vi "isr_ESP32.vi"() -> (7 "SenalFuga":bool)   [LabVIEW 2019]
uses:
  <vilib>/myRIO/Instrument Drivers/Onboard IO/DIO/typedefs/DIO Reference.ctl
  <vilib>/myRIO/Common/Instrument Driver Framework/Utilities/typedefs/myRIO Generic Hardware Reference.ctl
  <vilib>/myRIO/Common/Instrument Driver Framework/Utilities/typedefs/Hardware Version Enum.ctl
  <vilib>/myRIO/Common/Instrument Driver Framework/Utilities/typedefs/myRIO v1.0 Reference.ctl
  <vilib>/myRIO/Common/Instrument Driver Framework/Utilities/typedefs/Generic FPGA Reference.ctl
  <vilib>/myRIO/Common/Instrument Driver Framework/myRIO v1.0/DIO/typedefs/DIO Channels List.ctl
  <vilib>/myRIO/Common/Instrument Driver Framework/myRIO v1.0/DIO/typedefs/DIO Channels Enum.ctl
  <vilib>/userDefined/High Color/nirio_resource_hc.ctl
  <vilib>/myRIO/Common/Instrument Driver Framework/Utilities/vis/Is FPGA Ref Available.vi
  <vilib>/myRIO/Common/Instrument Driver Framework/myRIO v1.0/DIO/vis/myRIO v1.1 Open DIO.vi
  <vilib>/myRIO/Instrument Drivers/Onboard IO/DIO/vis/Read.vi
  <vilib>/myRIO/Common/Instrument Driver Framework/Utilities/vis/Validate Channels.vi
  <vilib>/myRIO/Common/Instrument Driver Framework/myRIO v1.0/DIO/vis/myRIO v1.0 Reserve DIO.vi
  <vilib>/myRIO/Common/Instrument Driver Framework/myRIO v1.0/Resource Manager/vis/myRIO v1.0 Reserve Channel List.vi
  <vilib>/myRIO/Common/Instrument Driver Framework/myRIO v1.0/DIO/vis/myRIO v1.0 Build MUX Configuration DIO.vi
  <vilib>/myRIO/Common/Instrument Driver Framework/myRIO v1.0/Resource Manager/vis/myRIO v1.0 Reserve Channel.vi
  <vilib>/myRIO/Common/Instrument Driver Framework/myRIO v1.0/Resource Manager/vis/myRIO v1.0 Unreserve Channel.vi
  <vilib>/myRIO/Common/Instrument Driver Framework/myRIO v1.0/Resource Manager/vis/myRIO v1.0 Create Configuration List.vi
  <vilib>/myRIO/Common/Instrument Driver Framework/myRIO v1.0/Resource Manager/vis/myRIO v1.0 Build Mutex Name.vi
  <vilib>/Utility/VariantDataType/GetNumericInfo.vi
  <vilib>/Utility/error.llb/Error Cluster From Error Code.vi
  <vilib>/myRIO/Common/Instrument Driver Framework/myRIO v1.0/myRIO v1.1 Open.vi
  <vilib>/myRIO/Common/Instrument Driver Framework/Utilities/vis/IO Manager.vi
  <vilib>/myRIO/Common/Instrument Driver Framework/Utilities/vis/Configuration Manager.vi
  <vilib>/myRIO/Common/Instrument Driver Framework/myRIO v1.0/Resource Manager/vis/myRIO v1.0 Configure IO.vi
  <vilib>/myRIO/Common/Instrument Driver Framework/myRIO v1.0/myRIO v1.0 Close.vi
  <vilib>/myRIO/Common/Instrument Driver Framework/myRIO v1.0/DIO/vis/myRIO v1.0 Read DIO.vi
  <vilib>/myRIO/Express VI/Onboard IO/DI/DI Express VI.xnode
  <vilib>/myRIO/Instrument Drivers/Onboard IO/DIO/vis/myRIO DIO Open.xnode
  <vilib>/myRIO/Instrument Drivers/Onboard IO/DIO/DIO.lvlib
panel:
  in  "Test_MIC4":bool
  out "FugaEn_MIC4":bool
  in  "Test_MIC5":bool
  out "FugaEn_MIC5":bool
  in  "Test_MIC6":bool
  out "FugaEn_MIC6":bool
  in  "Test_MIC3":bool
  out "FugaEn_MIC3":bool
  in  "Test_MIC2":bool
  out "FugaEn_MIC2":bool
  out "FugaEn_MIC1":bool
  in  "Test_MIC1":bool
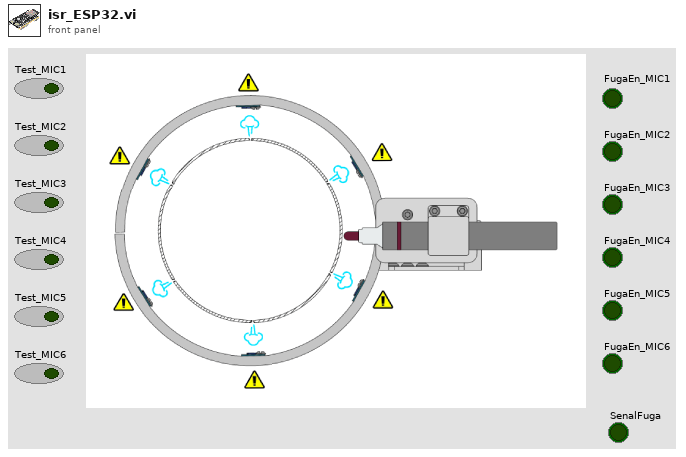
[diagram p1: front panel]
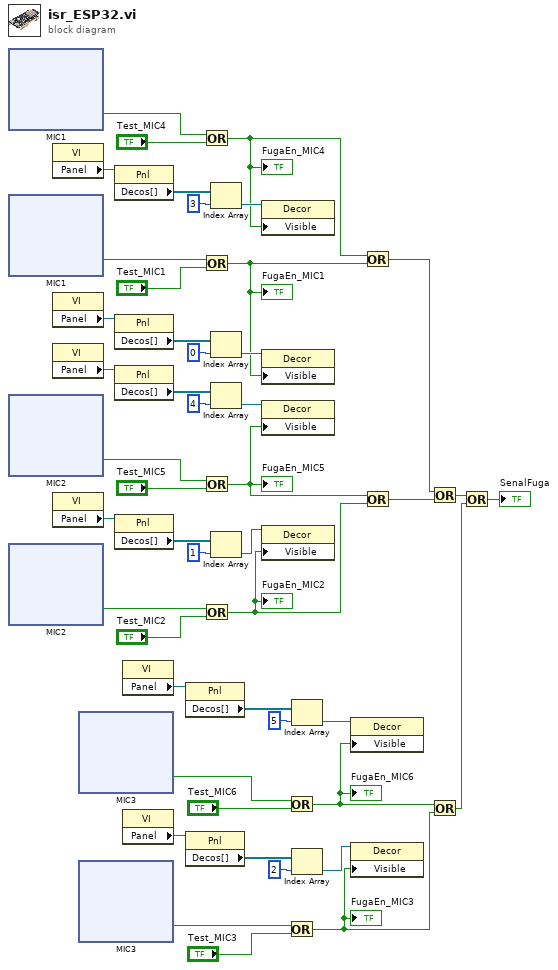
[diagram p0: block diagram]
diagram:
  n1 = xnode ("MIC1")() -> ("B/DIO3 (Pin 17)"=w38:bool)  [unwired: 1 in, 1 out]
  n2 = xnode ("MIC1")() -> ("B/DIO0 (Pin 11)"=w47:bool)  [unwired: 1 in, 1 out]
  n3 = xnode ("MIC2")() -> ("B/DIO4 (Pin 19)"=w37:bool)  [unwired: 1 in, 1 out]
  n4 = xnode ("MIC2")() -> ("B/DIO1 (Pin 13)"=w44:bool)  [unwired: 1 in, 1 out]
  n5 = property class="VI"() -> ("Panel"=w35:refnum<vi>)  [unwired: 2 in, 2 out]
  n6 = property class="VI"() -> ("Panel"=w28:refnum<vi>)  [unwired: 2 in, 2 out]
  n7 = property class="VI"() -> ("Panel"=w27:refnum<vi>)  [unwired: 2 in, 2 out]
  n8 = property class="VI"() -> ("Panel"=w20:refnum<vi>)  [unwired: 2 in, 2 out]
  n9 = xnode ("MIC3")() -> ("B/DIO5 (Pin 21)"=w36:bool)  [unwired: 1 in, 1 out]
  n10 = xnode ("MIC3")() -> ("B/DIO2 (Pin 15)"=w42:bool)  [unwired: 1 in, 1 out]
  n11 = property class="Pnl"(reference=w35) -> ("Decos[]"=w34:refnum<vi>[])  [unwired: 1 in, 2 out]
  n12 = property class="Pnl"(reference=w28) -> ("Decos[]"=w29:refnum<vi>[])  [unwired: 1 in, 2 out]
  n13 = property class="Pnl"(reference=w27) -> ("Decos[]"=w26:refnum<vi>[])  [unwired: 1 in, 2 out]
  n14 = property class="Pnl"(reference=w20) -> ("Decos[]"=w21:refnum<vi>[])  [unwired: 1 in, 2 out]
  n15 = property class="VI"() -> ("Panel"=w19:refnum<vi>)  [unwired: 2 in, 2 out]
  n16 = property class="VI"() -> ("Panel"=w12:refnum<vi>)  [unwired: 2 in, 2 out]
  n17 = property class="Pnl"(reference=w19) -> ("Decos[]"=w18:refnum<vi>[])  [unwired: 1 in, 2 out]
  n18 = property class="Pnl"(reference=w12) -> ("Decos[]"=w13:refnum<vi>[])  [unwired: 1 in, 2 out]
  n19 = Or(x=w38, y="Test_MIC4") -> (x .or. y?=w6:bool)
  "FugaEn_MIC4" <- w6
  n20 = Or(x=w47, y="Test_MIC1") -> (x .or. y?=w5:bool)
  "FugaEn_MIC1" <- w5
  n21 = Or(x=w37, y="Test_MIC5") -> (x .or. y?=w4:bool)
  "FugaEn_MIC5" <- w4
  n22 = Or(x=w44, y="Test_MIC2") -> (x .or. y?=w3:bool)
  "FugaEn_MIC2" <- w3
  n23 = Index Array(array=w34, index=3) -> (element=w33:refnum<vi>)
  n24 = Index Array(array=w29, index=0) -> (element=w30:refnum<vi>)
  n25 = Index Array(array=w26, index=4) -> (element=w25:refnum<vi>)
  n26 = Index Array(array=w21, index=1) -> (element=w22:refnum<vi>)
  n27 = property class="Decor"(reference=w33, "Visible"=w6) -> ()  [unwired: 1 in, 2 out]
  n28 = property class="Decor"(reference=w30, "Visible"=w5) -> ()  [unwired: 1 in, 2 out]
  n29 = property class="Decor"(reference=w25, "Visible"=w4) -> ()  [unwired: 1 in, 2 out]
  n30 = property class="Decor"(reference=w22, "Visible"=w3) -> ()  [unwired: 1 in, 2 out]
  n31 = Or(x=w36, y="Test_MIC6") -> (x .or. y?=w2:bool)
  "FugaEn_MIC6" <- w2
  n32 = Or(x=w42, y="Test_MIC3") -> (x .or. y?=w1:bool)
  "FugaEn_MIC3" <- w1
  n33 = Index Array(array=w18, index=5) -> (element=w17:refnum<vi>)
  n34 = Index Array(array=w13, index=2) -> (element=w14:refnum<vi>)
  n35 = property class="Decor"(reference=w17, "Visible"=w2) -> ()  [unwired: 1 in, 2 out]
  n36 = property class="Decor"(reference=w14, "Visible"=w1) -> ()  [unwired: 1 in, 2 out]
  n37 = Or(x=w6, y=w5) -> (x .or. y?=w10:bool)
  n38 = Or(x=w4, y=w3) -> (x .or. y?=w9:bool)
  n39 = Or(x=w10, y=w9) -> (x .or. y?=w8:bool)
  n40 = Or(x=w2, y=w1) -> (x .or. y?=w7:bool)
  n41 = Or(x=w8, y=w7) -> (x .or. y?=→"SenalFuga":bool)
